vi "Get VI Info.vi"(8 "error in (no error)":errorcluster, 11 "VI Path in":path) -> (0 "error out":errorcluster, 3 "VI Info out":T2)   [LabVIEW 2024, in "VI Info.lvlib"]
uses:
  VI Info.lvlib
  <vilib>/picture/picture.llb/imagedata.ctl
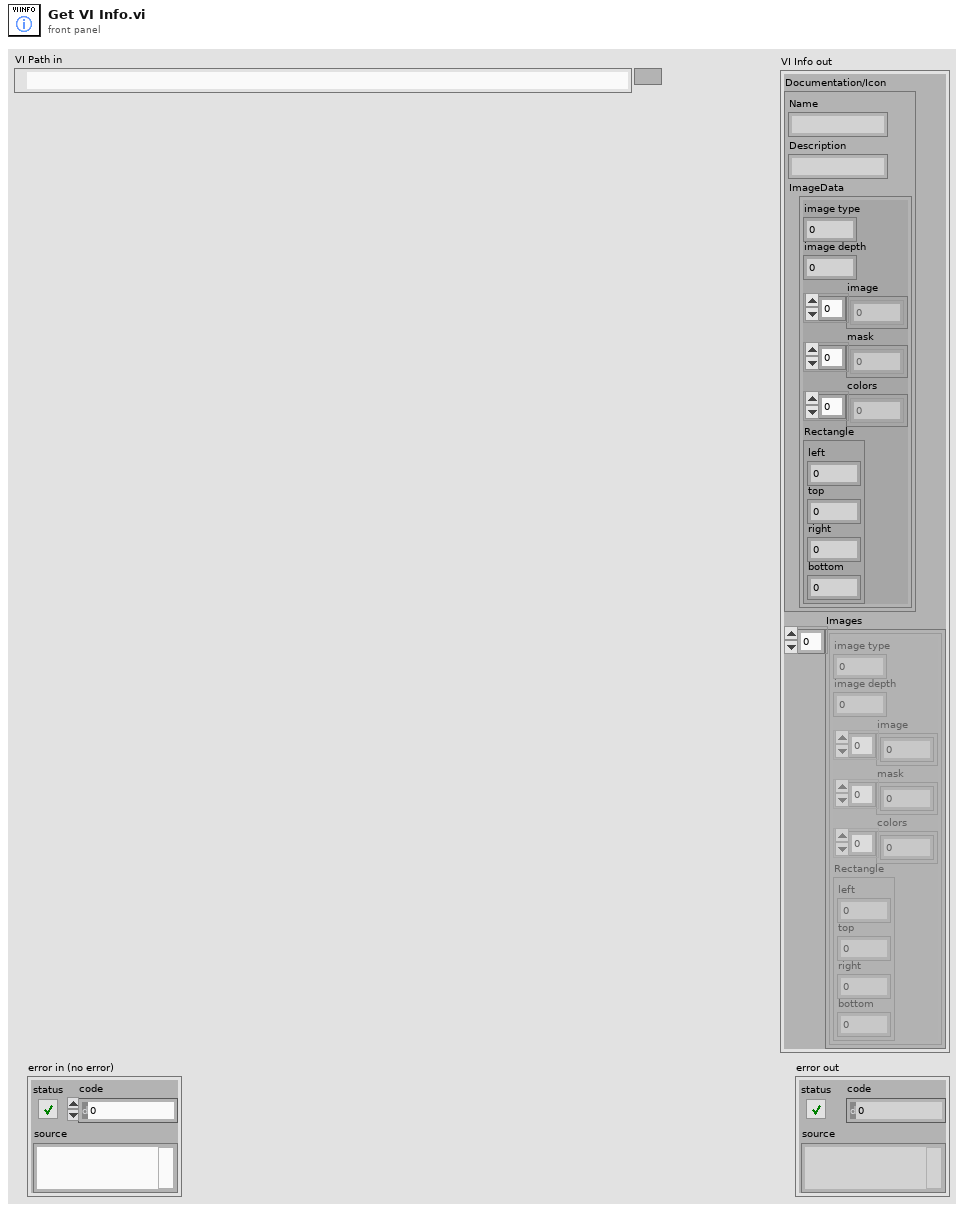
[diagram p1: front panel]
types:
  T1 = typedef "imagedata.ctl" = cluster{"image type":i32, "image depth":i32, "image":u8[], "mask":u8[], "colors":u32[], "Rectangle":cluster{"left":i16, "top":i16, "right":i16, "bottom":i16}}
  T2 = cluster{"Documentation/Icon":cluster{"Name":string, "Description":string, "ImageData":T1}, "Images":T1[]}
  T3 = cluster{cluster{"Left":i32, "Top":i32, "Right":u32, "Bottom":u32}, "SubDiag Label.Text":string, "Image Data":T1, "ClassName":string, refnum<vi>, "UID":i32}[]
  T4 = cluster{"Name":string, "Description":string, "ImageData":T1}
  T5 = cluster{"GObject":refnum<vi>, "Owner":refnum<vi>, "Numeric":dbl}[]
  T6 = cluster{"left":i16, "top":i16, "right":i16, "bottom":i16}
  T7 = cluster{"Rectangle":cluster{"left":i16, "top":i16, "right":i16, "bottom":i16}, string, "Block Diagram":T1, string, "TopLevelDiagram":refnum<vi>, "TLD UID":i32}
  T8 = cluster{"Rectangle":cluster{"Left":i32, "Top":i32, "Right":u32, "Bottom":u32}, "SubDiag Label.Text":string, "Image Data":T1, "ClassName":string, "My Refnum":refnum<vi>, "UID":i32, "Owner UID":i32, "Indexes of Children":i32[]}[]
  T9 = cluster{"Documentation/Icon":cluster{"Name":string, "Description":string, "ImageData":T1}, "Uncompressed Images":T1[]}
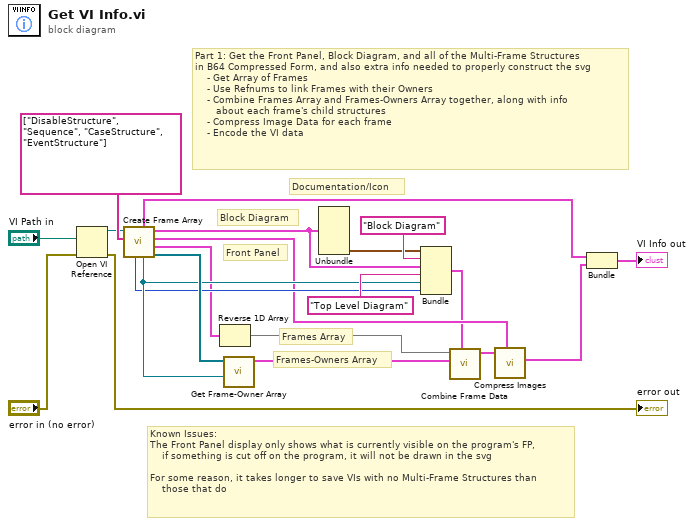
[diagram p0: block diagram]
diagram:
  # "Documentation/Icon"
  # "Frames-Owners Array"
  # "Frames Array"
  # "Block Diagram"
  # "Front Panel"
  # "Part 1: Get the Front Panel, Block Diagram, and all of the Multi-Frame Structures \nin B64 Compressed Form, and also extra info needed to properly construct the svg\n    - Get Array of Frames\n    - Use Refnums to link Frames with their Owners\n    - Combine Frames Array and Frames-Owners Array together, along with info\n       about each frame's child structures\n    - Compress Image Data for each frame\n    - Encode the VI data"
  # "Known Issues:\nThe Front Panel display only shows what is currently visible on the program's FP,\n    if something is cut off on the program, it will not be drawn in the svg\n\nFor some reason, it takes longer to save VIs with no Multi-Frame Structures than\n    those that do"
  n1 = Open VI Reference(vi path="VI Path in", error in (no error)="error in (no error)") -> (vi reference=w14:refnum<vi>, error out=→"error out":errorcluster)  [unwired: 4 in]
  n2 = call "Create Frame Array.vi"("Multi-Frame\nStructures"=string[] ["DisableStructure", "Sequence", "CaseStructure", "EventStructure"] ("Array"), "Refnum"=w14) -> ("Output References Array"=w18:refnum<vi>[], "Output Frame Array"=w9:T3, "Front Panel"=w10:T1, "Block Diagram"=w15:T1, "TopLevelDiagram"=w17:refnum<vi>, "Documentation/Icon"=w6:T4, "TLD UID"=w16:i32)  [unwired: 3 in]
  n3 = Reverse 1D Array(array=w9) -> (reversed array=w8:T3)
  n4 = call "Get Frame-Owner Array.vi"("Diagram"=w17, "References"=w18) -> ("Frames-Owners"=w12:T5)  [unwired: 9 in]
  n5 = Unbundle(w15) -> ("Rectangle"=w13:T6)  [unwired: 5 out]
  n6 = Bundle("Rectangle"=w13, "Block Diagram", "Block Diagram"=w15, "Top Level Diagram", "TopLevelDiagram"=w17, "TLD UID"=w16) -> (w5:T7)  [unwired: 1 in]
  n7 = call "Combine Frame Data.vi"("Block Diagram"=w5, "Frames-Owners"=w12, "Frames Array"=w8) -> ("Frame Data"=w11:T8)  [unwired: 8 in]
  n8 = call "Compress Images.vi"("Front Panel"=w10, "Frame Data"=w11) -> ("Uncompressed Images"=w2:T1[])  [unwired: 9 in]
  n9 = Bundle("Documentation/Icon"=w6, "Uncompressed Images"=w2) -> (→"VI Info out":T9)  [unwired: 1 in]
